vi "MAG3110_Init.vi"(3 "error in (no error)":errorcluster) -> (7 "VISA resource name out":refnum<visa-resource-name>="COM5", 10 "error out":errorcluster={"status"=FALSE, "code"=1073676294, "source"="VISA Read in MAG3110_Init.vi"})   [LabVIEW 2012]
uses:
  <vilib>/Instr/_visa.llb/VISA Configure Serial Port (Instr).vi
panel:
  in  "delay before read (ms)":u32=150
  out "read string":string
  out "bytes read":u32=374
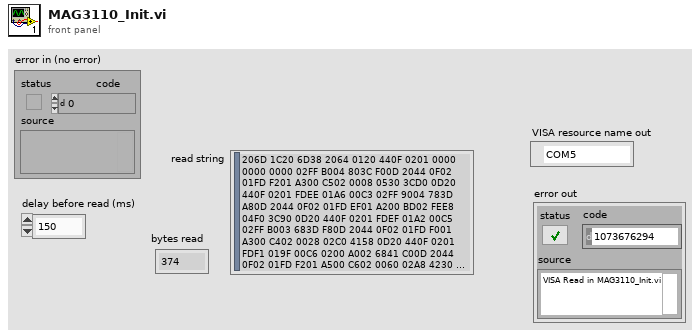
[diagram p1: front panel]
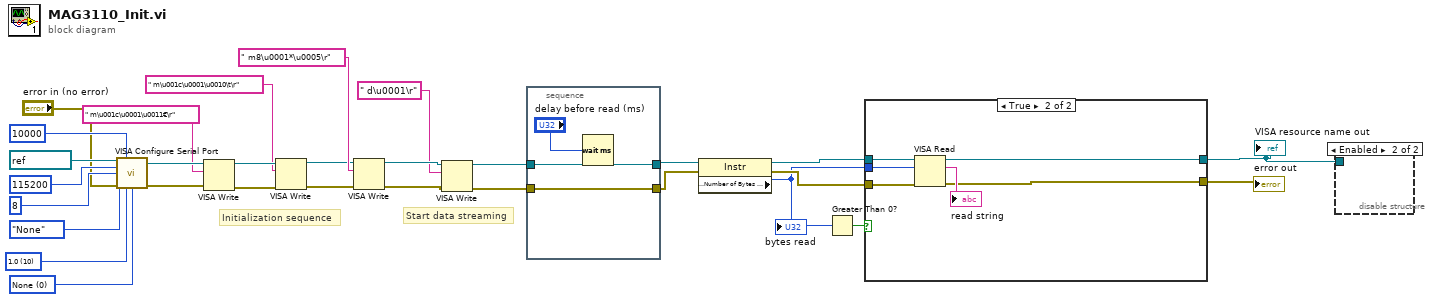
[diagram p0: block diagram]
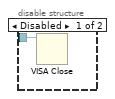
[diagram p2: hidden frame]
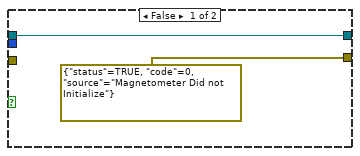
[diagram p3: hidden frame]
diagram:
  w24 = u16 0 items=["None", "XON/XOFF", "RTS/CTS", "XON/XOFF & RTS/CTS", "DTR/DSR", "XON/XOFF & DTR/DSR"] ("flow control (0:none)")
  w25 = u16 10 items=["1.0"=10, "1.5"=15, "2.0"=20] ("stop bits (10: 1 bit)")
  # "Start data streaming"
  # "Initialization sequence"
  n1 = call-poly "VISA Configure Serial Port"("VISA resource name"=refnum<visa-resource-name> "COM5", "timeout (10sec)"=u32 10000, "baud rate (9600)"=u32 115200, "data bits (8)"=u16 8, "parity (0:none)"=enum16{"None", "Odd", "Even", "Mark", "Space"}."None", "error in (no error)"="error in (no error)", "stop bits (10: 1 bit)"=w25, "flow control (0:none)"=w24) -> ("VISA resource name out"=w19:refnum<visa-resource-name>, "error out"=w23:errorcluster)  [unwired: 1 in, 5 out]
  n2 = VISA Write(VISA resource name=w19, write buffer=" m\u001c\u0001\u0011€\r", error in (no error)=w23) -> (VISA resource name out=w22:refnum<visa-resource-name>, error out=w21:errorcluster)  [unwired: 1 out]
  n3 = VISA Write(VISA resource name=w22, write buffer=" m\u001c\u0001\u0010\t\r", error in (no error)=w21) -> (VISA resource name out=w15:refnum<visa-resource-name>, error out=w20:errorcluster)  [unwired: 1 out]
  n4 = VISA Write(VISA resource name=w15, write buffer=" m8\u0001*\u0005\r", error in (no error)=w20) -> (VISA resource name out=w12:refnum<visa-resource-name>, error out=w11:errorcluster)  [unwired: 1 out]
  n5 = VISA Write(VISA resource name=w12, write buffer=" d\u0001\r", error in (no error)=w11) -> (VISA resource name out=w9:refnum<visa-resource-name>, error out=w8:errorcluster)  [unwired: 1 out]
  n6 = stacked-sequence {
    tunnel: w9 -> [w31]
    tunnel: [w32] -> w7
    tunnel: w8 -> [w32]
    tunnel: [w31] -> w6
    frame #0 {
      n7 = Wait (ms)(milliseconds to wait="delay before read (ms)") -> ()  [unwired: 1 out]
    }
  }
  n8 = property class="Instr"(reference=w6, error in=w7) -> (reference out=w14:refnum<visa-resource-name>, error out=w13:errorcluster, "Serial Settings:Number of Bytes at Serial Port"=w4:u32)
  "bytes read" <- w4
  n9 = Greater Than 0?(x=w4) -> (x > 0?=w3:bool)
  n10 = case shown="True" w3 {
    tunnel: w14 -> [w34 w41]
    tunnel: w13 -> [_ w40]
    tunnel: w4 -> [_ w38]
    tunnel: [w34 w37] -> w1
    tunnel: [errorcluster {"status"=TRUE, "code"=0, "source"="Magnetometer Did not Initialize"} ("error constant") w36] -> w2
    frame False {
    }
    frame True {
      n11 = VISA Read(VISA resource name=w41, byte count=w38, error in (no error)=w40) -> (VISA resource name out=w37:refnum<visa-resource-name>, read buffer=→"read string":string, error out=w36:errorcluster)  [unwired: 1 out]
    }
  }
  "error out" <- w2
  "VISA resource name out" <- w1
  n12 = disable-structure shown="Enabled" {
    disable-tunnel: w1 -> [w42 _]
    frame Disabled {
      n13 = VISA Close(VISA resource name=w42) -> ()  [unwired: 1 in, 1 out]
    }
    frame Enabled {
    }
  }
